vi "Helmholtz2D_FEM_Assemble_Prepare Triangle.vi"(9 "Y":dbl[](array[numeric]), 10 "X":dbl[](array[numeric]), 11 "Triangle In":i32[](array[numeric])) -> (0 "area":dbl, 1 "Tri Y":dbl[](array[numeric]), 2 "Tri X":dbl[](array[numeric]), 3 "Triangle Out":i32[](array[numeric]))   [LabVIEW 2020, in "NI_PDE.lvlib"]
uses:
  <vilib>/gmath/NI_PDE.lvlib
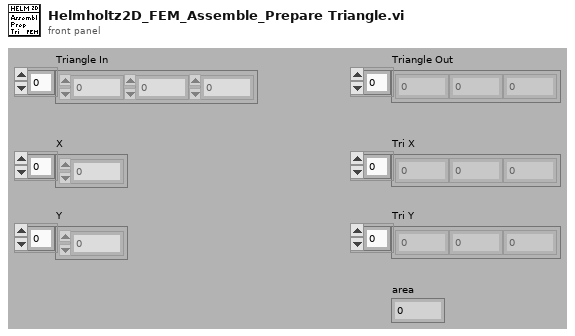
[diagram p1: front panel]
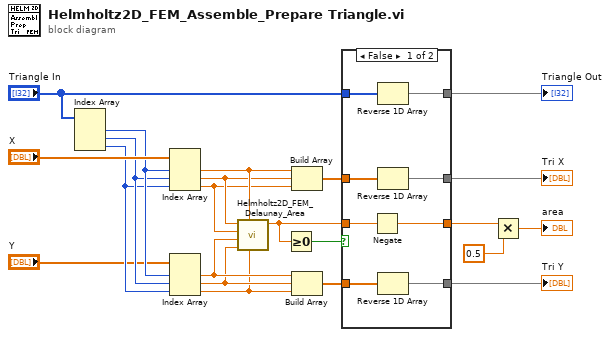
[diagram p0: block diagram]
diagram:
  n1 = Index Array(array="Triangle In") -> (element #1=w21:i32, element #2=w20:i32, element #3=w19:i32)  [unwired: 3 in]
  n2 = Index Array(array="X", index #1=w21, index #2=w20, index #3=w19) -> (element #1=w15:dbl, element #2=w14:dbl, element #3=w13:dbl)
  n3 = Index Array(array="Y", index #1=w21, index #2=w20, index #3=w19) -> (element #1=w12:dbl, element #2=w11:dbl, element #3=w10:dbl)
  n4 = call <vilib>:"Helmholtz2D_FEM_Delaunay_Area.vi"("y3"=w10, "x1"=w15, "y2"=w11, "y1"=w12, "x3"=w13, "x2"=w14) -> ("area"=w16:dbl)  [unwired: 5 out]
  n5 = Greater Or Equal To 0?(x=w16) -> (x >= 0?=w17:bool)
  n6 = Build Array(w15, w14, w13) -> (w8:dbl[])
  n7 = Build Array(w12, w11, w10) -> (w7:dbl[])
  n8 = case shown="False" w17 {
    tunnel: w16 -> [w24 w31]
    tunnel: "Triangle In" -> [w30 w34]
    tunnel: w8 -> [w28 w33]
    tunnel: w7 -> [w26 w32]
    tunnel: [w29 w34] -> w6
    tunnel: [w27 w33] -> w5
    tunnel: [w25 w32] -> w4
    tunnel: [w23 w31] -> w3
    frame False {
      n9 = Negate(x=w24) -> (-x=w23:dbl)
      n10 = Reverse 1D Array(array=w30) -> (reversed array=w29:i32[])
      n11 = Reverse 1D Array(array=w28) -> (reversed array=w27:dbl[])
      n12 = Reverse 1D Array(array=w26) -> (reversed array=w25:dbl[])
    }
    frame True {
    }
  }
  "Triangle Out" <- w6
  "Tri X" <- w5
  "Tri Y" <- w4
  n13 = Multiply(x=w3, y=0.5) -> (x*y=→"area":dbl)
